vi "FB_Enable.vi"(8 "error in":errorcluster, 11 "VISA Refnum in":refnum<visa-resource-name>) -> (0 "error out":errorcluster, 2 "Reply":string, 3 "VISA Refnum out":refnum<visa-resource-name>)   [LabVIEW 2017]
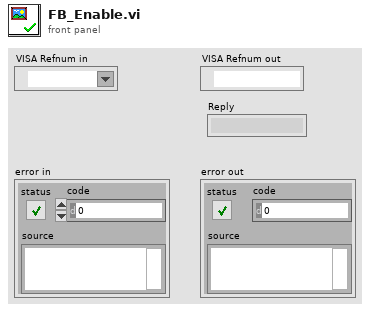
[diagram p1: front panel]
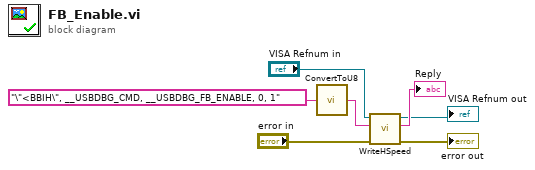
[diagram p0: block diagram]
diagram:
  n1 = call <userlib>:"ConvertToU8.vi"("struct"="\"<BBIH\", __USBDBG_CMD, __USBDBG_FB_ENABLE, 0, 1" ("write buffer")) -> ("Binary"=w3:string)
  n2 = call <userlib>:"WriteHSpeed.vi"("error in"="error in", "write buffer"=w3, "VISA Refnum in"="VISA Refnum in") -> ("error out"=→"error out":errorcluster, "read buffer"=→"Reply":string, "VISA Refnum out"=→"VISA Refnum out":refnum<visa-resource-name>)  [unwired: 6 in]
